vi "SeCrTs-Data reader from shared variable.vi"(0 "Data in":string, 3 "empty?":bool, 5 "error IO":errorcluster) -> (19 "error out":errorcluster)   [LabVIEW 2022 SP3]
uses:
  91644d88-8a3a-46f6-9314-183f243c8ec6.vi
  3d41d14a-1e81-4e0e-8a5a-4fdd32b6dd05.vi
  Globals/SeCrTS-DD globals.vi
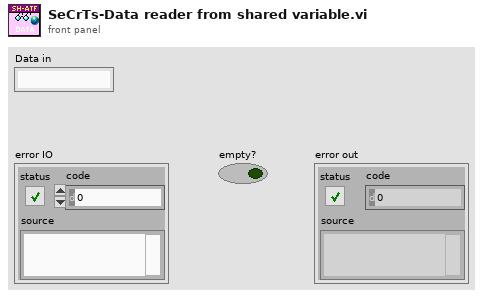
[diagram p1: front panel]
types:
  T1 = cluster{"C/NC":bool, "Start/Stop Log":bool[], "Log Name":string, "Config":cluster{"AO config":cluster{"Channel_Name":string, "Channel_Number":string, "Default_Value":dbl, "Units":string}[], "AI config":cluster{"Channel_Name":string, "Channel_Number":string, "Pre_Scale_min":dbl, "Pre_Scale_max":dbl, "Sensor_min":dbl, "Sensor_max":dbl, "Units":string}[], "DI config":cluster{"Channel_Name":string, "Channel_Number":string, "Default_Value":bool, "DI invert?":bool}[], "DO config":cluster{"Channel_Name":string, "Channel_Number":string, "Default_Value":bool, "DO invert?":bool}[], "TC config":cluster{"Channel_Name":string, "Channel_Number":string, "Pre_Scale_min":dbl, "Pre_Scale_max":dbl, "units":i32, " type":i32}[], "ACC config":cluster{"Channel_Name":string, "Channel_Number":string, "Pre_Scale_min":dbl, "Pre_Scale_max":dbl, "Terminal configuration":i32, "Sensitivity":dbl, "Sensitivity units":i32}[], "SG config":cluster{"Channel_Name":string, "Channel_Number":string, "Pre_Scale_min":dbl, "Pre_Scale_max":dbl}[], "Strain Gauge Settings":cluster{"poisson ratio":dbl, "nominal gage resistance":dbl, "gage factor":dbl}, "Bridge Settings":cluster{"voltage excitation value":dbl, "voltage excitation source":i32, "initial bridge voltage":dbl, "lead wire resistance":dbl, "strain configuration":i32}, "Sample Rate":cluster{"AI Sample Rate":dbl[], "AO Sample Rate":dbl[], "DI Sample Rate":dbl[], "TC Sample Rate":dbl[], "DO Sample Rate":dbl[], "SG Sample Rate":dbl[], "ACC Sample Rate":dbl[]}}, "Log min":dbl, "Drive":cluster{"Drive_Health":bool, "Drive_Frequency":u32, "Drive_Status":bool, "Drive_RPM":u32, "Drive_Direction":bool, "Acceleration state":bool, "Steady state":bool, "Deceleration state":bool, "Drive_Enable":bool, "Drive set_RPM":dbl}, "HOLD UPDATE":bool}
  T2 = cluster{"AO config":cluster{"Channel_Name":string, "Channel_Number":string, "Default_Value":dbl, "Units":string}[], "AI config":cluster{"Channel_Name":string, "Channel_Number":string, "Pre_Scale_min":dbl, "Pre_Scale_max":dbl, "Sensor_min":dbl, "Sensor_max":dbl, "Units":string}[], "DI config":cluster{"Channel_Name":string, "Channel_Number":string, "Default_Value":bool, "DI invert?":bool}[], "DO config":cluster{"Channel_Name":string, "Channel_Number":string, "Default_Value":bool, "DO invert?":bool}[], "TC config":cluster{"Channel_Name":string, "Channel_Number":string, "Pre_Scale_min":dbl, "Pre_Scale_max":dbl, "units":i32, " type":i32}[], "ACC config":cluster{"Channel_Name":string, "Channel_Number":string, "Pre_Scale_min":dbl, "Pre_Scale_max":dbl, "Terminal configuration":i32, "Sensitivity":dbl, "Sensitivity units":i32}[], "SG config":cluster{"Channel_Name":string, "Channel_Number":string, "Pre_Scale_min":dbl, "Pre_Scale_max":dbl}[], "Strain Gauge Settings":cluster{"poisson ratio":dbl, "nominal gage resistance":dbl, "gage factor":dbl}, "Bridge Settings":cluster{"voltage excitation value":dbl, "voltage excitation source":i32, "initial bridge voltage":dbl, "lead wire resistance":dbl, "strain configuration":i32}, "Sample Rate":cluster{"AI Sample Rate":dbl[], "AO Sample Rate":dbl[], "DI Sample Rate":dbl[], "TC Sample Rate":dbl[], "DO Sample Rate":dbl[], "SG Sample Rate":dbl[], "ACC Sample Rate":dbl[]}}
  T3 = cluster{"Drive_Health":bool, "Drive_Frequency":u32, "Drive_Status":bool, "Drive_RPM":u32, "Drive_Direction":bool, "Acceleration state":bool, "Steady state":bool, "Deceleration state":bool, "Drive_Enable":bool, "Drive set_RPM":dbl}
  T4 = cluster{"Channel names":cluster{"AI_C_Data P":string[], "AI_V_Data P":string[], "AO_Data P":string[], "DO_Data P":string[], "ACC_Data P":string[], "TC Data P":string[], "Drive_A_C":string[], "Drive_A_D":string[], "AI_C_Data S":string[], "DO_Data S":string[]}, "DI Names":cluster{"Di P":string[], "Di S":string[]}}
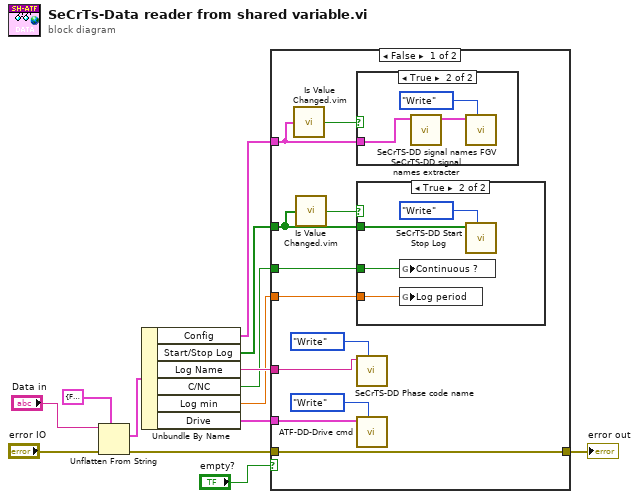
[diagram p0: block diagram]
diagram:
  n1 = Unflatten From String(type=T1 {"C/NC"=FALSE, "Start/Stop Log"=[], "Log Name"="", "Config"={"AO config"=[], "AI config"=[], "DI config"=[], "DO config"=[], "TC config"=[], "ACC config"=[], "SG config"=[], "Strain Gauge Settings"={"poisson ratio"=0.0, "nominal gage resistance"=0.0, "gage factor"=0.0}, "Bridge Settings"={"voltage excitation value"=0.0, "voltage excitation source"=0, "initial bridge voltage"=0.0, "lead wire resistance"=0.0, "strain configuration"=0}, "Sample Rate"={"AI Sample Rate"=[], "AO Sample Rate"=[], "DI Sample Rate"=[], "TC Sample Rate"=[], "DO Sample Rate"=[], "SG Sample Rate"=[], "ACC Sample Rate"=[]}}, "Log min"=0.0, "Drive"={"Drive_Health"=FALSE, "Drive_Frequency"=0, "Drive_Status"=FALSE, "Drive_RPM"=0, "Drive_Direction"=FALSE, "Acceleration state"=FALSE, "Steady state"=FALSE, "Deceleration state"=FALSE, "Drive_Enable"=FALSE, "Drive set_RPM"=0.0}, "HOLD UPDATE"=FALSE} ("notification"), binary string="Data in", error in (no error)="error IO") -> (value=w11:T1, error out=w3:errorcluster)  [unwired: 2 in, 1 out]
  n2 = Unbundle By Name(w11) -> ("Config"=w9:T2, "Start/Stop Log"=w8:bool[], "Log Name"=w7:string, "C/NC"=w6:bool, "Log min"=w5:dbl, "Drive"=w4:T3)
  n3 = case shown="False" "empty?" {
    tunnel: w7 -> [w23 _]
    tunnel: w9 -> [w20 _]
    tunnel: w8 -> [w19 _]
    tunnel: w3 -> [w18 w32]
    tunnel: [w18 w32] -> w12
    tunnel: w6 -> [w17 _]
    tunnel: w5 -> [w16 _]
    tunnel: w4 -> [w14 _]
    frame False {
      n4 = call "Is Value Changed.vim"("value"=w20) -> ("changed or first call?"=w22:bool)
      n5 = call "Is Value Changed.vim"("value"=w19) -> ("changed or first call?"=w21:bool)
      n6 = case shown="True" w22 {
        tunnel: w20 -> [_ w31]
        frame False {
        }
        frame True {
          n7 = call "SeCrTS-DD signal names extracter.vi"("input cluster"=w31) -> ("Signal names"=w30:T4)  [unwired: 10 in]
          n8 = call "SeCrTS-DD signal names FGV.vi"("Enum"=enum16{"Read", "Write"}."Write", "Signal names"=w30) -> ()  [unwired: 8 in, 2 out]
        }
      }
      n9 = case shown="True" w21 {
        tunnel: w19 -> [_ w27]
        tunnel: w17 -> [_ w25]
        tunnel: w16 -> [_ w26]
        frame False {
        }
        frame True {
          n10 = global write "SeCrTS-DD globals.vi" "Continuous ?"(w25) -> ()
          n11 = global write "SeCrTS-DD globals.vi" "Log period"(w26) -> ()
          n12 = call "SeCrTS-DD Start Stop Log.vi"("Enum"=enum16{"Read", "Write"}."Write", "Start Stop log"=w27) -> ()  [unwired: 8 in, 2 out]
        }
      }
      n13 = call "SeCrTS-DD Phase code name.vi"("Enum"=enum16{"Read", "Write"}."Write", "Phase code W"=w23) -> ()  [unwired: 8 in, 2 out]
      n14 = call "ATF-DD-Drive cmd.vi"("Enum"=enum16{"Read", "Write"}."Write", "Data.Drive"=w14) -> ()  [unwired: 8 in, 2 out]
    }
    frame True {
    }
  }
  "error out" <- w12
